vi "Clear Math Calculation Test Failures .vi"(8 "error in (no error)":errorcluster, 10 "Limit Number (0: Limit1)":i32(ring) items=["Limit1", "Limit2"], 11 "VISA resource name":refnum<visa-resource-name>) -> (0 "error out":errorcluster, 3 "VISA resource name out":refnum<visa-resource-name>)   [LabVIEW 2020, in "Keithley 6517.lvlib"]
doc: "Clears the Limit1 and Limit2 test failures for CALC 3 math calculation. \n\nNote:\nA failure is also cleared when the limit test is disabled that can be configured by <b>Configure Limit Test.vi</b>.\n\nThis VI is <B>NOT</B> compatible with model <B>6514</B>."
uses:
  <instrlib>/Keithley 6517/Keithley 6517.lvlib
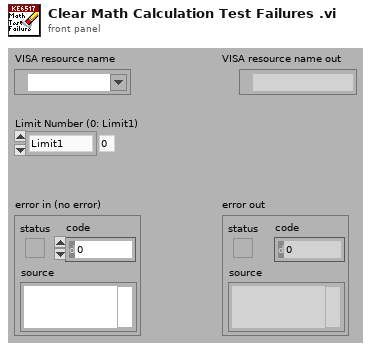
[diagram p1: front panel]
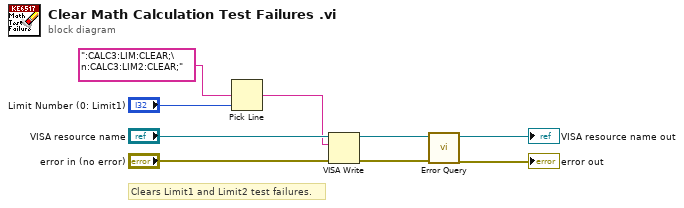
[diagram p0: block diagram]
diagram:
  # "Clears Limit1 and Limit2 test failures."
  n1 = Pick Line(multi-line string=":CALC3:LIM:CLEAR;\n:CALC3:LIM2:CLEAR;", line index="Limit Number (0: Limit1)") -> (output string=w1:string)  [unwired: 1 in]
  n2 = VISA Write(VISA resource name="VISA resource name", write buffer=w1, error in (no error)="error in (no error)") -> (VISA resource name out=w7:refnum<visa-resource-name>, error out=w6:errorcluster)  [unwired: 1 out]
  n3 = call <instrlib>:"Error Query.vi"("error in (no error)"=w6, "VISA resource name"=w7) -> ("error out"=→"error out":errorcluster, "VISA resource name out"=→"VISA resource name out":refnum<visa-resource-name>)  [unwired: 6 in, 2 out]
